vi "RPC Method Invoke.vi"(8 "error in (no error)":errorcluster, 11 "OOP Server in":refnum<class "Query Server.lvclass">) -> (0 "error out":errorcluster, 3 "OOP Server out":refnum<class "Query Server.lvclass">)   [LabVIEW 2019, in "Query Server.lvlib" / "Query Server.lvclass"]
uses:
  Query Server.lvclass
  Query Server.lvclass/Query Server.ctl
  RPC Messages/InvokeResponse/InvokeResponse_Data.ctl
  typeDefs/Server Internal Message.ctl
panel:
  out "Data":string
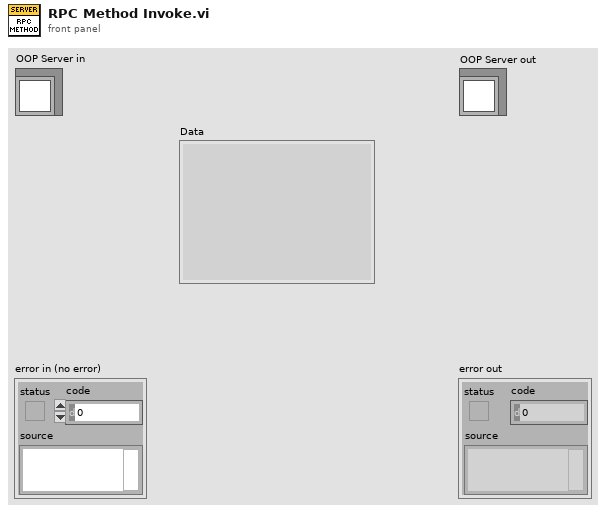
[diagram p1: front panel]
types:
  T1 = typedef "Query Server.lvlib/Query Server.lvclass/InvokeResponse_Data.ctl" = cluster{"status":i32}
  T2 = typedef "Query Server.lvlib/Query Server.lvclass/Server Internal Message.ctl" = cluster{"Command":string, "Data":variant}
  T3 = typedef "Query Server.lvlib/Query Server.lvclass/Server Internal UEs.ctl" = cluster{"Invoke Internal UE":refnum<user-event>, "Query Internal UE":refnum<user-event>, "Register Internal UE":refnum<user-event>}
  T4 = typedef "Query Server.lvlib/Query Server.lvclass/Server gRPC UEs.ctl" = cluster{"Invoke gRPC UE":refnum<user-event>, "Query gRPC UE":refnum<user-event>, "Register gRPC UE":refnum<user-event>}
  T5 = typedef "Query Server.lvlib/gprc-lvsupport.lvlib/grpcId.ctl" = u64
  T6 = typedef "Query Server.lvlib/Query Server.lvclass/InvokeRequest_Data.ctl" = cluster{"command":string, "parameter":string}
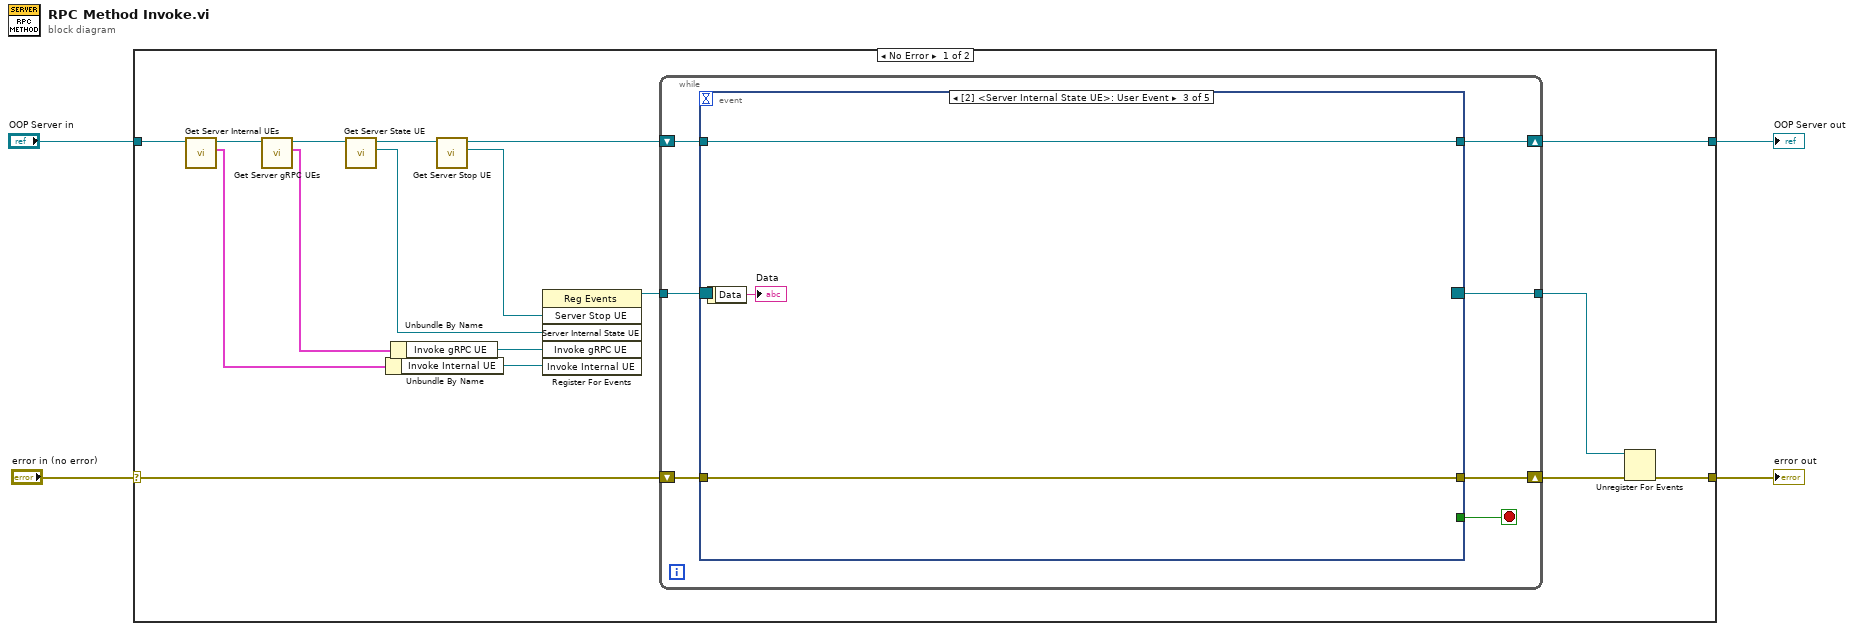
[diagram p0: block diagram]
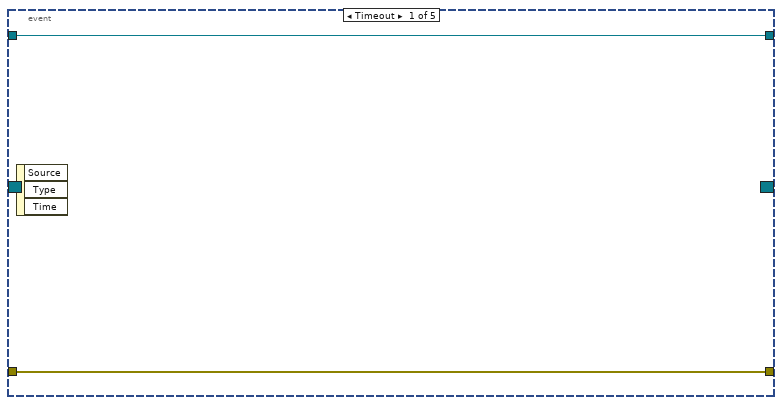
[diagram p2: hidden frame]
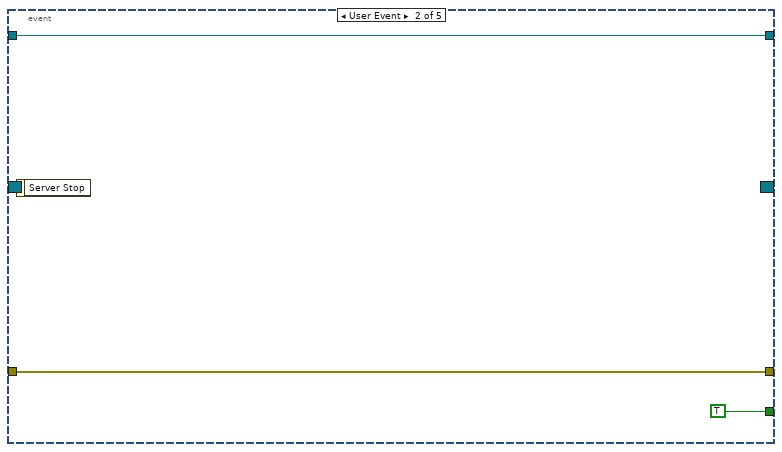
[diagram p3: hidden frame]
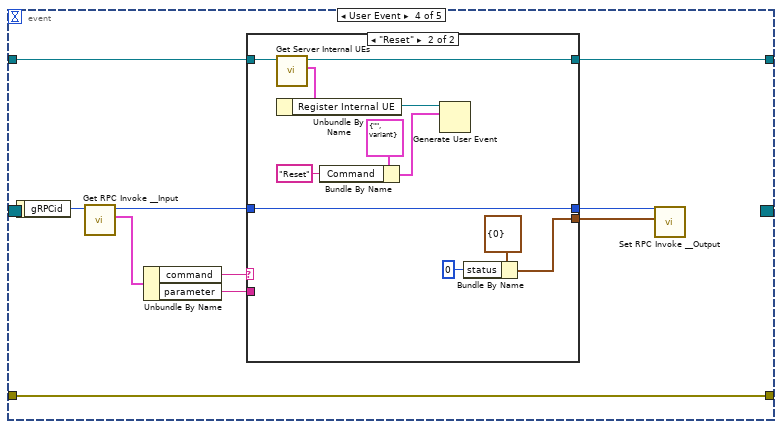
[diagram p4: hidden frame]
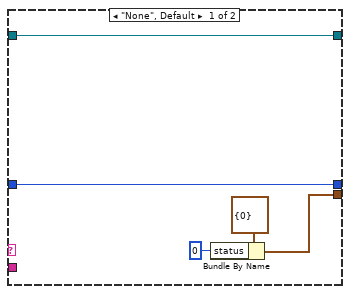
[diagram p5: hidden frame]
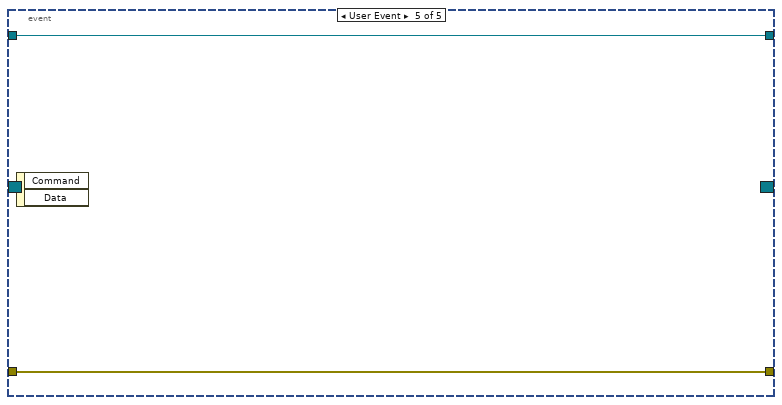
[diagram p6: hidden frame]
diagram:
  n1 = case shown="No Error" "error in (no error)" {
    selector: "error in (no error)" -> [w17 w66]
    tunnel: [w15 w66] -> w3
    tunnel: "OOP Server in" -> [w19 w65]
    tunnel: [w5 w65] -> w1
    frame No Error {
      n2 = call "Get Server Internal UEs.vi"("OOP Server in"=w19) -> ("Server Internal UEs"=w11:T3, "OOP Server out"=w18:refnum<class "Query Server.lvclass">)  [unwired: 9 in]
      n3 = call "Get Server gRPC UEs.vi"("OOP Server in"=w18) -> ("Server gRPC UEs"=w13:T4, "OOP Server out"=w8:refnum<class "Query Server.lvclass">)  [unwired: 9 in]
      n4 = call "Get Server State UE.vi"("Template Server in"=w8) -> ("Server Internal State UE"=w6:refnum<user-event>, "Template Server out"=w7:refnum<class "Query Server.lvclass">)  [unwired: 9 in]
      n5 = Unbundle By Name ("Unbundle Internal UE")(w11) -> ("Invoke Internal UE"=w10:refnum<user-event>)
      n6 = Unbundle By Name ("Unbundle gRPC UE")(w13) -> ("Invoke gRPC UE"=w12:refnum<user-event>)
      n7 = call "Get Server Stop UE.vi"("OOP Server in"=w7) -> ("Server Stop UE"=w21:refnum<user-event>, "OOP Server out"=w9:refnum<class "Query Server.lvclass">)  [unwired: 9 in]
      n8 = register-events(w21, w6, w12, w10) -> (reference out=w20:refnum<event-registration>)  [unwired: 2 in, 1 out]
      n9 = while {
        tunnel: w20 -> [w28]
        tunnel: [w24] -> w14
        shift-right: [w25] -> w16
        shift-left: w17 -> [w26]
        shift-right: [w22] -> w5
        shift-left: w9 -> [w23]
        stop <- w27 stop-if-true
        n10 = event "RPC Method Event Structure" shown="[2] <Server Internal State UE>: User Event" {
          selector: w28 -> [_ _ _ _ _]
          dyn-events: [_ _ _ _ _] -> w24
          timeout: _ -> [_ _ _ _ _]
          tunnel: [_ TRUE _ _ _] -> w27
          tunnel: w26 -> [w30 w32 w36 w46 w64]
          tunnel: [w30 w32 w36 w46 w64] -> w25
          tunnel: w23 -> [w29 w31 w35 w41 w63]
          tunnel: [w29 w31 w35 w40 w63] -> w22
          event Timeout {
            n11 = event-data() -> ()  [unwired: 1 in, 3 out]
          }
          event User Event {
            n12 = event-data() -> ()  [unwired: 1 in, 1 out]
          }
          event User Event {
            n13 = event-data() -> ("Data"=→"Data":string)  [unwired: 1 in]
          }
          event User Event {
            n14 = event-data() -> ("gRPCid"=w45:T5)  [unwired: 1 in]
            n15 = call "Get RPC Invoke __Input.vi"("gRPCid in"=w45) -> ("Message Data"=w44:T6, "gRPCid out"=w39:T5)  [unwired: 8 in, 1 out]
            n16 = Unbundle By Name(w44) -> ("command"=w43:string, "parameter"=w42:string)
            n17 = case shown="\"Reset\"" w43 {
              tunnel: w42 -> [_ _]
              tunnel: w41 -> [w51 w62]
              tunnel: [w51 w56] -> w40
              tunnel: w39 -> [w49 w55]
              tunnel: [w49 w55] -> w38
              tunnel: [w48 w52] -> w37
              frame "None", Default {
                n18 = Bundle By Name(cluster=T1 {"status"=0} ("Message Data"), "status"=0) -> (w48:T1)
              }
              frame "Reset" {
                n19 = call "Get Server Internal UEs.vi"("OOP Server in"=w62) -> ("Server Internal UEs"=w61:T3, "OOP Server out"=w56:refnum<class "Query Server.lvclass">)  [unwired: 9 in]
                n20 = Unbundle By Name(w61) -> ("Register Internal UE"=w60:refnum<user-event>)
                n21 = Bundle By Name(cluster=T2 {"Command"="", "Data"=variant} ("event data"), "Command"="Reset") -> (w57:T2)
                n22 = Generate User Event(user event=w60, event data cluster=w57) -> ()  [unwired: 2 in, 2 out]
                n23 = Bundle By Name(cluster=T1 {"status"=0} ("Message Data"), "status"=0) -> (w52:T1)
              }
            }
            n24 = call "Set RPC Invoke __Output.vi"("Message Data"=w37, "gRPCid in"=w38) -> ()  [unwired: 9 in, 1 out]
          }
          event User Event {
            n25 = event-data() -> ()  [unwired: 1 in, 2 out]
          }
        }
      }
      n26 = Unregister For Events(event registration refnum=w14, error in=w16) -> (error out=w15:errorcluster)
    }
    frame Error {
    }
  }
  "error out" <- w3
  "OOP Server out" <- w1
